vi "UART Receive.vi"(0 "I/O In":T1, 7 "Baud Rate (9600)":u32=9600) -> (15 "Dout":u8)   [LabVIEW 2012, in "UART 8N1 (FPGA).lvlib"]
uses:
  UART 8N1 (FPGA).lvlib
  RxD CMD.ctl
  <vilib>/Platform/TimedLoop/XDataNode/wakeup.ctl
  <vilib>/Platform/TimedLoop/XDataNode/XDNodeRunTimeDep.lvlib
  <vilib>/Platform/TimedLoop/XDataNode/nitl_modes.ctl
  <vilib>/Platform/TimedLoop/XDataNode/timing_clust.ctl
  <vilib>/Platform/TimedLoop/XDataNode/XDataNode.xnode
  <vilib>/eio/EIONode/EIONode.xnode
  <vilib>/rvi/DataTransferAndStorage/Container/XNode/niFpgaContainer.xnode
  <vilib>/rvi/FIFO/Fifo_Resource/niFpgaFifoEmulationRefIn.vi
  <vilib>/rvi/DataTransferAndStorage/Register/Emulation/niFpgaRegisterEmulationRefIn.vi
  <vilib>/rvi/eio/common/nirviEmuTemplateMethod_errors.vi
panel:
  out "Receive Buffer Overflow":bool
  # "UART Receive\nRxD, 8N1"
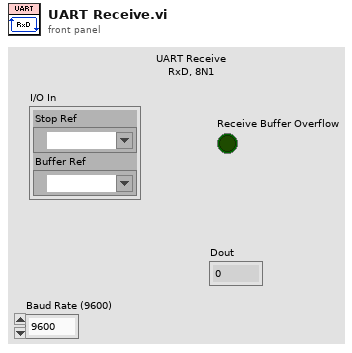
[diagram p1: front panel]
types:
  T1 = cluster{"Stop Ref":refnum<k21>, "Buffer Ref":refnum<k21>}
  T2 = typedef "UART 8N1 (FPGA).lvlib/RxD CMD.ctl" = enum16{"Init", "Wait on Falling Edge", "Wait Half Bit", "Wait One Bit", "Read Data Bit", "Wait Stop Time", "Close"}
  T3 = typedef "XDNodeRunTimeDep.lvlib/timing_clust.ctl" = cluster{"Expected End [f-1]":u64, "Actual End [f-1]":u64, "Finished Late? [f-1]":bool, "Expected End [i-1]":u64, "Actual End [i-1]":u64, "Finished Late? [i-1]":bool, "Expected Start [i]":u64, "Actual Start [i]":u64, "Expected Start [f]":u64, "Actual Start [f]":u64, "Source Name":string, "Structure Name":string, "Period":i64, "Deadline":i64, "Offset":i64, "Start":i64, "Priority":i32, "Timeout":i32, "Mode":T4, "Wakeup Reason":T5, "Error":errorcluster, "Source Type":string, "Secondary Source Type":string, "Global End Time":u64, "Global Start Time":u64, "Frame Duration":u64, "Iteration Duration":u64, "Assigned CPU":i32, "I/O Scan Engine Mode":u32}
  T4 = typedef "XDNodeRunTimeDep.lvlib/nitl_modes.ctl" = enum32{"No Change", "Process missed periods, maintain original phase", "Discard missed periods, maintain original phase", "Process missed periods, ignore original phase", "Discard missed periods, ignore original phase"}
  T5 = typedef "XDNodeRunTimeDep.lvlib/wakeup.ctl" = enum32{"Normal", "Aborted", "Asynchronous wakeup", "Timing source error", "Timed loop error", "Timeout"}
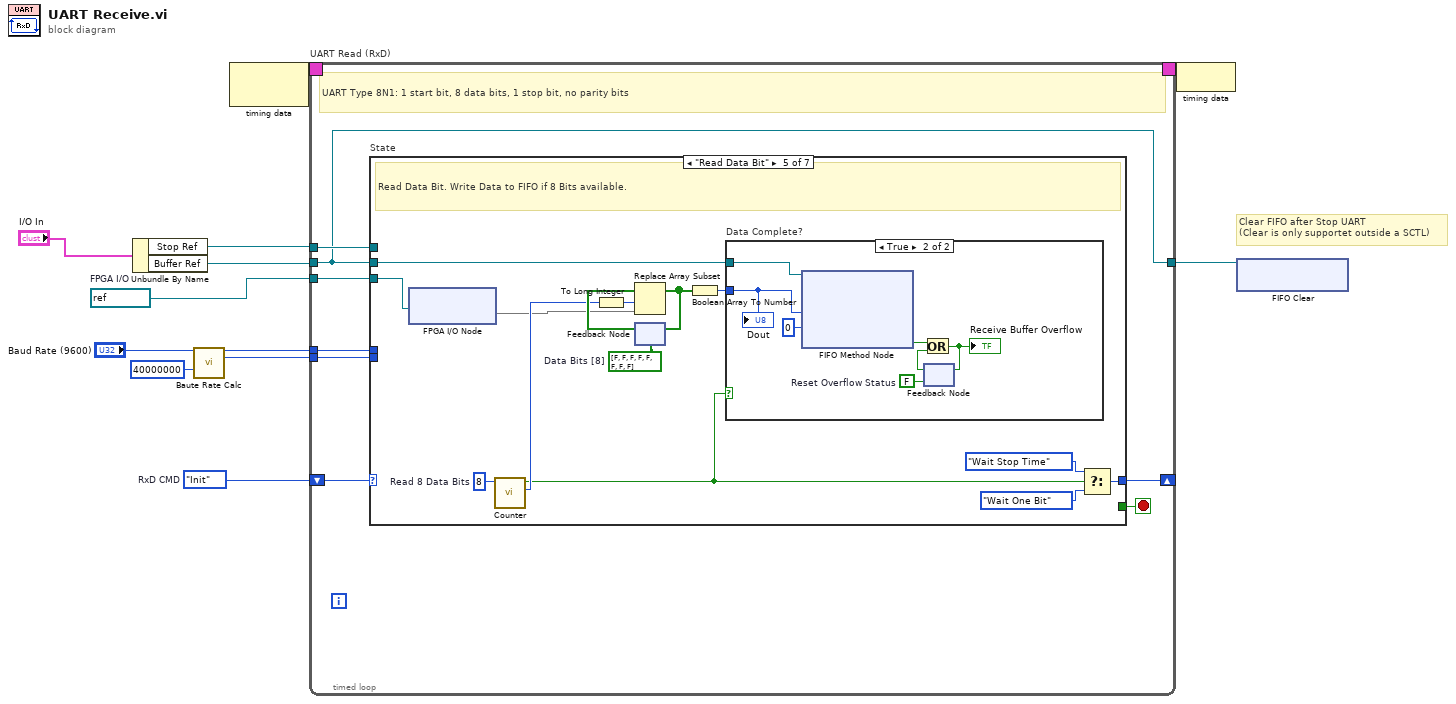
[diagram p0: block diagram]
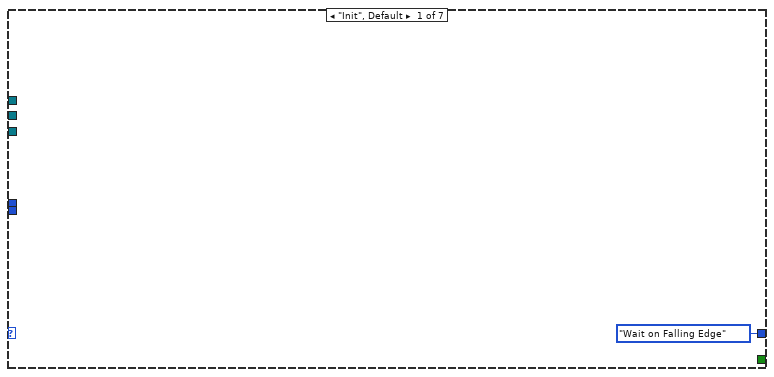
[diagram p2: hidden frame]
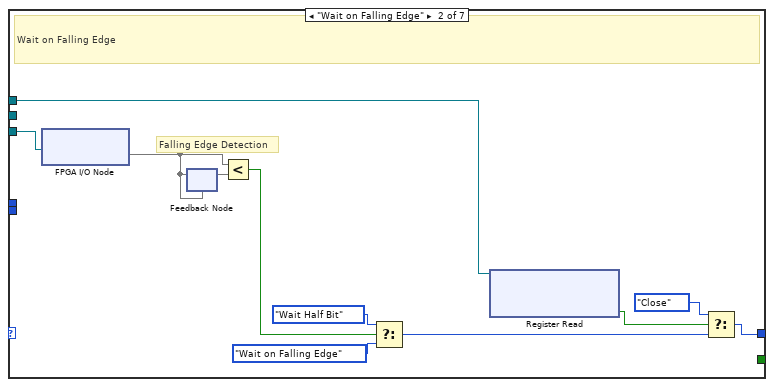
[diagram p3: hidden frame]
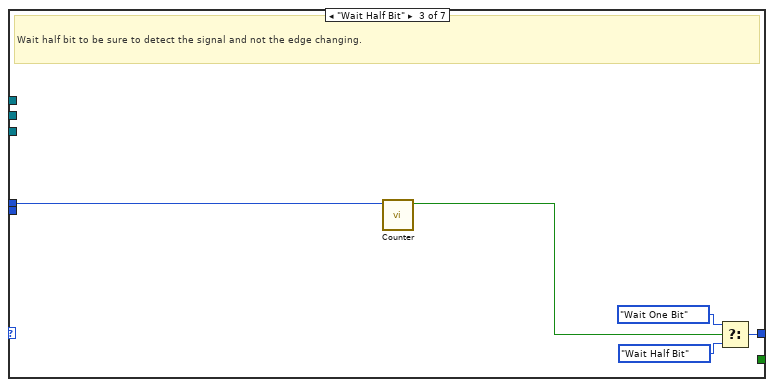
[diagram p4: hidden frame]
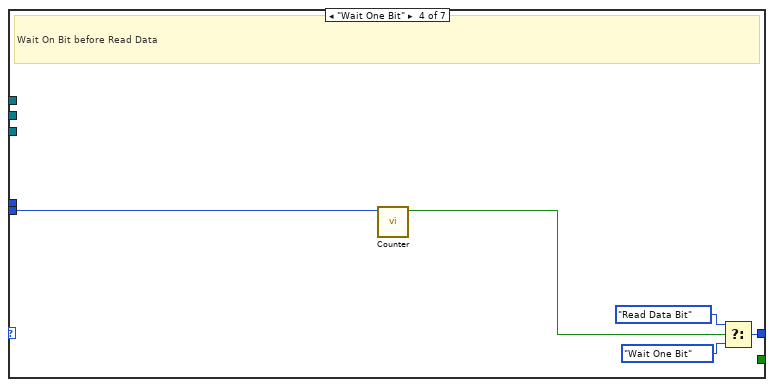
[diagram p5: hidden frame]
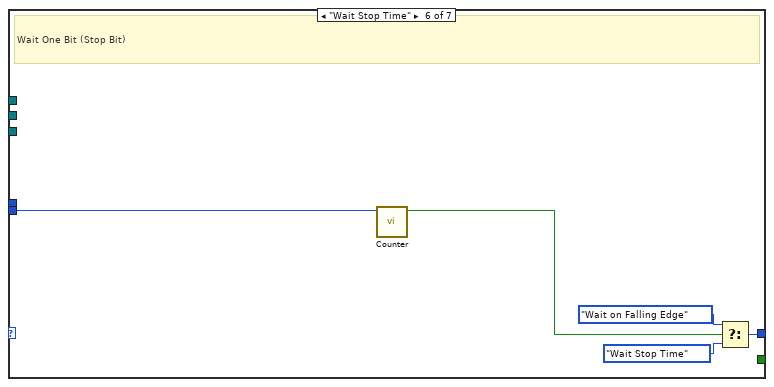
[diagram p7: hidden frame]
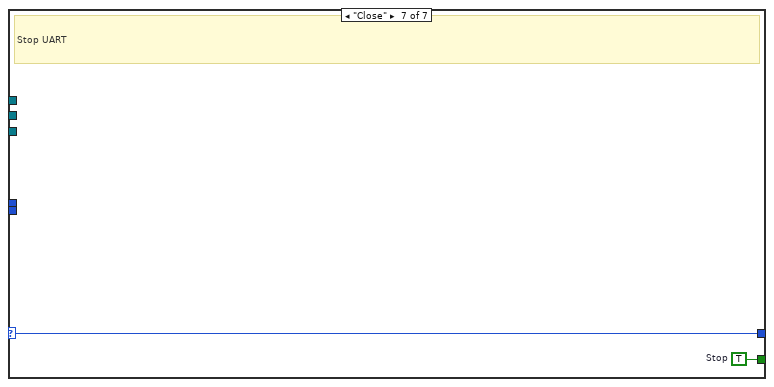
[diagram p8: hidden frame]
diagram:
  w3 = refnum<k21> "DIO25"  # FPGA I/O
  w10 = RxD_CMD."Init"  # RxD CMD
  # "Clear FIFO after Stop UART\n(Clear is only supportet outside a SCTL)"
  n1 = Unbundle By Name("I/O In") -> ("Stop Ref"=w2:refnum<k21>, "Buffer Ref"=w1:refnum<k21>)
  n2 = call "Baute Rate Calc.vi"("Baud Rate (9600)"="Baud Rate (9600)", "FPGA Clock Rate (40000000)"=u32 40000000) -> ("Half Bit"=w8:u32, "One Bit"=w7:u32)  [unwired: 10 in, 2 out]
  n3 = node-c288() -> (w12:T3)  [unwired: 1 in]
  n4 = timed-loop "UART Read (RxD)" {
    timing: w12 -> [_]
    timing-out: [_] -> w11
    shift-right: [w19] -> _
    shift-left: w10 -> [w16]
    tunnel: w8 -> [w18]
    tunnel: w7 -> [w17]
    tunnel: w1 -> [w14]
    tunnel: w2 -> [w15]
    tunnel: [w14] -> w9
    tunnel: w3 -> [w13]
    stop <- w20 stop-if-true
    # "UART Type 8N1: 1 start bit, 8 data bits, 1 stop bit, no parity bits"
    n5 = case "State" shown="\"Read Data Bit\"" w16 {
      selector: w16 -> [_ _ _ _ _ _ w69]
      tunnel: [_ _ _ _ _ _ w70] -> w20
      tunnel: [RxD_CMD."Wait on Falling Edge" ("RxD State") w28 w35 w39 w50 w65 w69] -> w19
      tunnel: w18 -> [_ _ w33 _ _ _ _]
      tunnel: w17 -> [_ _ _ w38 _ w64 _]
      tunnel: w14 -> [_ _ _ _ w45 _ _]
      tunnel: w15 -> [_ w27 _ _ _ _ _]
      tunnel: w13 -> [_ w22 _ _ w43 _ _]
      frame "Init", Default {
      }
      frame "Wait on Falling Edge" {
        # "Falling Edge Detection"
        # "Wait on Falling Edge"
        n6 = xnode "FPGA I/O Node"("FPGA I/O In"=w22) -> ("I/O Item"=w23)  [unwired: 1 out]
        n7 = feedback #1(w23) -> (w25)
        n8 = feedback-in #1(w23) -> ()
        n9 = Less?(x=w23, y=w25) -> (x < y?=w24:bool)
        n10 = Select(t=RxD_CMD."Wait Half Bit", s=w24, f=RxD_CMD."Wait on Falling Edge" ("RxD State")) -> (s? t:f=w29:T2)
        n11 = xnode ("Register Read")("Register In"=w27) -> ("Data"=w26:bool)  [unwired: 1 out]
        n12 = Select(t=RxD_CMD."Close", s=w26, f=w29) -> (s? t:f=w28:T2)
      }
      frame "Wait Half Bit" {
        # "Wait half bit to be sure to detect the signal and not the edge changing."
        n13 = call "Counter.vi"("Counter End  Value"=w33) -> ("End Reached"=w34:bool)  [unwired: 9 in, 1 out]
        n14 = Select(t=RxD_CMD."Wait One Bit", s=w34, f=RxD_CMD."Wait Half Bit" ("RxD State")) -> (s? t:f=w35:T2)
      }
      frame "Wait One Bit" {
        # "Wait On Bit before Read Data"
        n15 = call "Counter.vi"("Counter End  Value"=w38) -> ("End Reached"=w42:bool)  [unwired: 9 in, 1 out]
        n16 = Select(t=RxD_CMD."Read Data Bit", s=w42, f=RxD_CMD."Wait One Bit" ("RxD State")) -> (s? t:f=w39:T2)
      }
      frame "Read Data Bit" {
        w46 = u32 8  # Read 8 Data Bits
        w56 = bool[] [FALSE, FALSE, FALSE, FALSE, FALSE, FALSE, FALSE, FALSE]  # Data Bits [8]
        # "Read Data Bit. Write Data to FIFO if 8 Bits available."
        n17 = xnode "FPGA I/O Node"("FPGA I/O In"=w43) -> ("I/O Item"=w44)  [unwired: 1 out]
        n18 = call "Counter.vi"("Counter End  Value"=w46) -> ("Counter Value"=w54:u32, "End Reached"=w48:bool)  [unwired: 9 in]
        n19 = To Long Integer(number=w54) -> (32bit integer=w53:i32)
        n20 = feedback #2(w56) -> (w55:bool[])
        n21 = Replace Array Subset(array=w55, new element=w44, index=w53) -> (w49:bool[])
        n22 = feedback-in #2(w49) -> ()
        n23 = Boolean Array To Number(Boolean array=w49) -> (number=w47:u8)
        n24 = case "Data Complete?" shown="True" w48 {
          tunnel: w47 -> [_ w63]
          tunnel: w45 -> [_ w57]
          frame False {
          }
          frame True {
            w59 = FALSE  # Reset Overflow Status
            n25 = xnode ("FIFO Method Node")("Element"=w63, "Timeout"=0, "FIFO In"=w57) -> ("Timed Out?"=w62:bool)  [unwired: 1 out]
            n26 = feedback #3(w59) -> (w60:bool)
            n27 = Or(x=w62, y=w60) -> (x .or. y?=w61:bool)
            "Receive Buffer Overflow" <- w61
            n28 = feedback-in #3(w61) -> ()
            "Dout" <- w63
          }
        }
        n29 = Select(t=RxD_CMD."Wait Stop Time", s=w48, f=RxD_CMD."Wait One Bit" ("RxD State")) -> (s? t:f=w50:T2)
      }
      frame "Wait Stop Time" {
        # "Wait One Bit (Stop Bit)"
        n30 = call "Counter.vi"("Counter End  Value"=w64) -> ("End Reached"=w66:bool)  [unwired: 9 in, 1 out]
        n31 = Select(t=RxD_CMD."Wait on Falling Edge", s=w66, f=RxD_CMD."Wait Stop Time" ("RxD State")) -> (s? t:f=w65:T2)
      }
      frame "Close" {
        w70 = TRUE  # Stop
        # "Stop UART"
      }
    }
  }
  n32 = node-c288(w11) -> ()
  n33 = xnode ("FIFO Clear")("FIFO In"=w9) -> ()  [unwired: 1 out]
